vi "Global destination achieved.vi"() -> ()   [LabVIEW 2020]
panel:
  out "Global destination achieved":bool
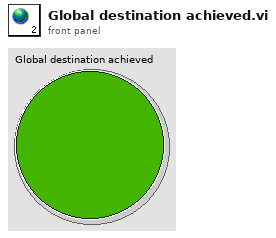
[diagram p1: front panel]
diagram:
